vi "WPI_RelayToDigitalModule.vi"(11 "RelayDevRef":T2={"DevStatus"={"status"=FALSE, "code"=0, "source"=""}, "Relay Channel"=enum."Relay 1", "Relay Direction"=enum."Both directions"}) -> (3 "DigitalModuleDevRef":T1)   [LabVIEW 2017]
doc: "This software is licensed. Open the labview\\readme\\WPI Robotics Library Open Source License.txt file for more information."
uses:
  <vilib>/Rock Robotics/WPI/Relay/WPI_RelayDevRef.ctl
  <vilib>/Rock Robotics/SystemInterfaces/DIO/FPGA_DIORelayChannel.ctl
  <vilib>/Rock Robotics/WPI/Relay/WPI_RelayDirection.ctl
  <vilib>/Rock Robotics/WPI/DigitalModule/WPI_DigitalModuleDeviceRef.ctl
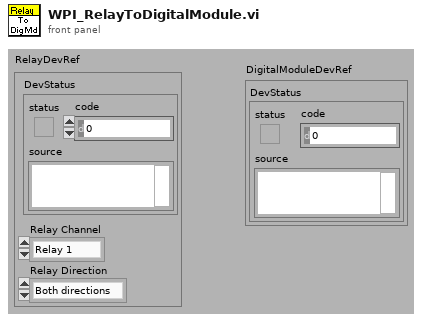
[diagram p1: front panel]
types:
  T1 = typedef "WPI_DigitalModuleDeviceRef.ctl" = cluster{"DevStatus":errorcluster}
  T2 = typedef "WPI_RelayDevRef.ctl" = cluster{"DevStatus":errorcluster, "Relay Channel":T3, "Relay Direction":T4}
  T3 = typedef "FPGA_DIORelayChannel.ctl" = enum8{"Relay 0", "Relay 1", "Relay 2", "Relay 3", "Invalid"}
  T4 = typedef "WPI_RelayDirection.ctl" = enum16{"Both directions", "Forward only", "Reverse only"}
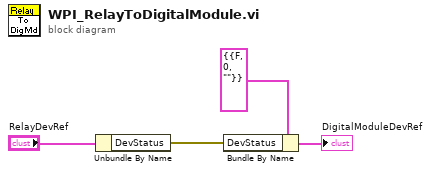
[diagram p0: block diagram]
diagram:
  n1 = Unbundle By Name("RelayDevRef") -> ("DevStatus"=w2:errorcluster)
  n2 = Bundle By Name(cluster=T1 {"DevStatus"={"status"=FALSE, "code"=0, "source"=""}} ("DigitalModuleDevRef"), "DevStatus"=w2) -> (→"DigitalModuleDevRef":T1)
